vi "NotARefNum.vi"(3 "reference in":refnum<class "IG#.lvclass">) -> (0 "not a refnum?":bool, 1 "reference out":refnum<class "IG#.lvclass">)   [LabVIEW 2020, in "IG#.lvclass"]
doc: "Checks if the specified object reference is valid."
uses:
  IG#.lvclass
panel:
  # "NOTICE -- YOU MUST LEAVE THIS NOTICE IN PLACE.  PER THE TERMS OF THE BSD LICENSE  (http://www.opensource.org/licenses/bsd-license.php).\nYOU MAY SUBLICENSE THIS SOFTWARE IN ANY WAY THAT DOES NOT CONFLICT WITH THIS LICENSE.\n\nCopyright (c) 2010, AddQ <http://www.addq.com>, Author: Mattias Ericsson <mattias.ericsson@addq.se>\n\nAll rights reserved."
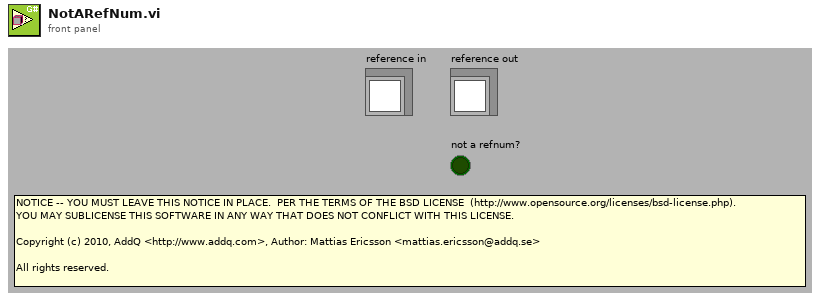
[diagram p1: front panel]
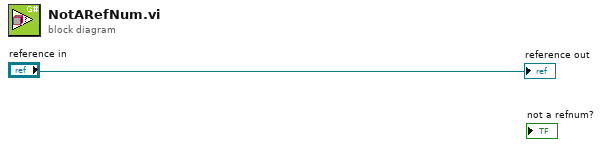
[diagram p0: block diagram]
diagram:
  "reference out" <- "reference in"
